vi "Reject Promise.vi"(8 "error in (no error)":errorcluster, 10 "Reason":errorcluster, 11 "Promise in":refnum<class "Promise.lvclass">) -> (0 "error out":errorcluster, 3 "Promise out":refnum<class "Promise.lvclass">)   [LabVIEW 2017, in "Promise.lvlib" / "Promise.lvclass"]
doc: "Cause any readers to error out with Reason."
uses:
  Promise.lvclass
  Rejected Promise/Rejected Promise.lvclass
  Rejected Promise/Rejected Promise.lvclass/Rejected Promise.ctl
  Promise.lvclass/Promise.ctl
  382b5372-11d9-45be-bc9b-e1bf09c8258a.vi
  Rejected Promise/Write Reason.vi
  Resolve Promise.vi
  <vilib>/Utility/error.llb/Error Cluster From Error Code.vi
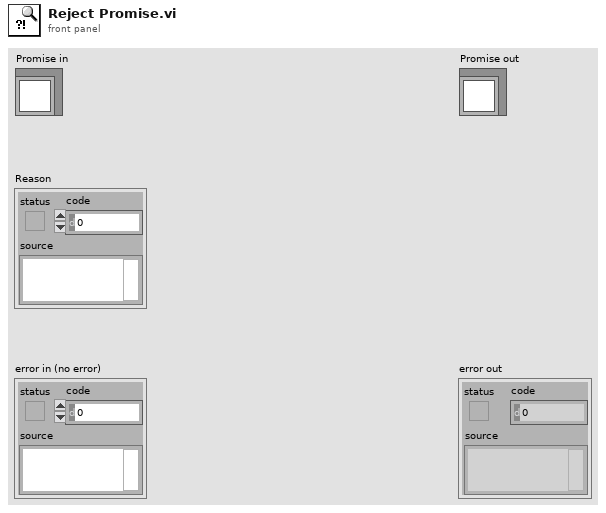
[diagram p1: front panel]
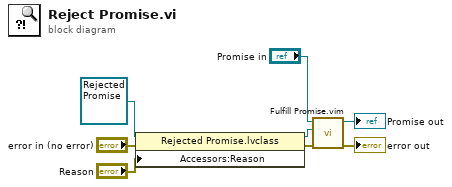
[diagram p0: block diagram]
diagram:
  n1 = property class="Rejected Promise.lvclass"(reference=refnum<class "Rejected Promise.lvclass"> refnum ("Future.lvlib:Rejected Future.lvclass"), error in="error in (no error)", "Accessors:Reason"="Reason") -> (reference out=w3:refnum<class "Rejected Promise.lvclass">, error out=w1:errorcluster)
  n2 = call "Fulfill Promise.vim"("error in (no error)"=w1, "Value"=w3, "Promise in"="Promise in") -> ("error out"=→"error out":errorcluster, "Promise out"=→"Promise out":refnum<class "Promise.lvclass">)  [unwired: 7 in]
